vi "PCIE-1810.vi"   [LabVIEW 2020]
uses:
  <userlib>/DAQNavi Polymorphic VI/create/DAQNavi Create Channel(AI-Voltage).vi
  Global_Variable/Global.vi
  <userlib>/DAQNavi Polymorphic VI/read/DAQNavi Read (Analog 1D DBL NChan 1Samp).vi
types:
  T1 = cluster{"输入轴扭矩":dbl, "输出轴扭矩小":dbl, "输出轴扭矩大":dbl, "吸收电流":dbl, "传感器电压":dbl}
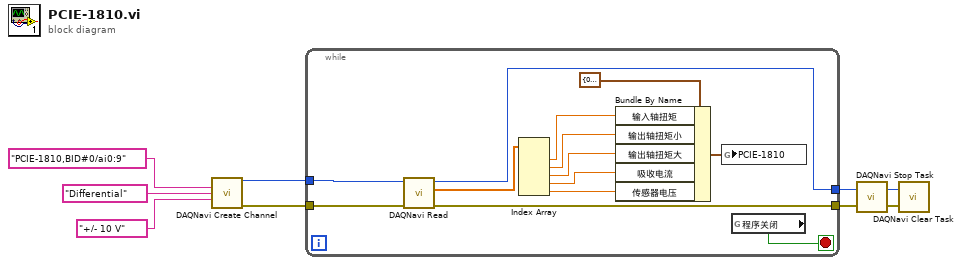
[diagram p0: block diagram]
diagram:
  n1 = call-poly <userlib>:"DAQNavi Create Channel.vi"("physical channels"="PCIE-1810,BID#0/ai0:9", "signal type"="Differential", "value range"="+/- 10 V") -> ("task out"=w6:i32, "error out"=w5:errorcluster)  [unwired: 11 in]
  n2 = while {
    tunnel: w5 -> [w21]
    tunnel: [w19] -> w3
    tunnel: w6 -> [w22]
    tunnel: [w20] -> w4
    stop <- w18 stop-if-true
    n3 = call-poly <userlib>:"DAQNavi Read.vi"("error in (no error)"=w21, "task in"=w22) -> ("error out"=w19:errorcluster, "data"=w17:dbl[], "task out"=w20:i32)  [unwired: 7 in]
    n4 = Index Array(array=w17) -> (element #1=w14:dbl, element #2=w13:dbl, element #3=w12:dbl, element #4=w11:dbl, element #5=w10:dbl)  [unwired: 5 in]
    n5 = Bundle By Name(cluster=T1 {"输入轴扭矩"=0.0, "输出轴扭矩小"=0.0, "输出轴扭矩大"=0.0, "吸收电流"=0.0, "传感器电压"=0.0} ("PCIE-1810"), "输入轴扭矩"=w14, "输出轴扭矩小"=w13, "输出轴扭矩大"=w12, "吸收电流"=w11, "传感器电压"=w10) -> (w15:T1)
    n6 = global write "Global.vi" "PCIE-1810"(w15) -> ()
    n7 = global read "Global.vi" "程序关闭"() -> (w18:bool)
  }
  n8 = call <userlib>:"DAQNavi Stop Task.vi"("error in (no error)"=w3, "task in"=w4) -> ("error out"=w1:errorcluster, "task out"=w2:i32)
  n9 = call <userlib>:"DAQNavi Clear Task.vi"("error in (no error)"=w1, "task in"=w2) -> ()  [unwired: 1 in, 1 out]
